vi "Wave Array Record LV2.vi"(2 "吸声测试结果IN":T1, 3 "W / R":enum16{"Write", "Read"}(ring)) -> (0 "吸声测试结果Out":T1)   [LabVIEW 2018]
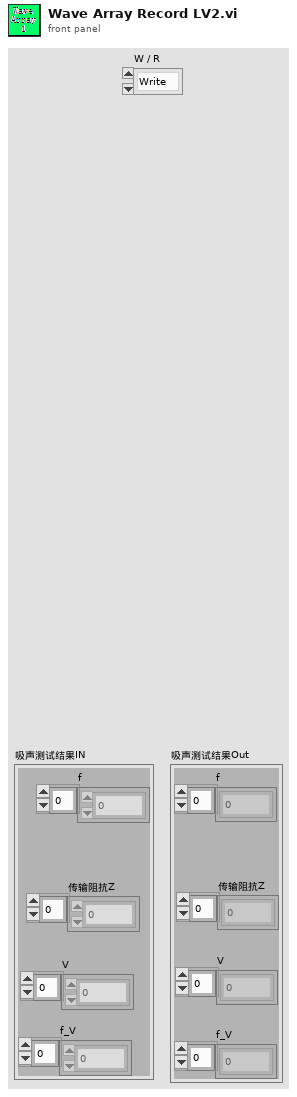
[diagram p1: front panel]
types:
  T1 = cluster{"f":dbl[], "传输阻抗Z":cdb[], "V":cdb[], "f_V":dbl[]}
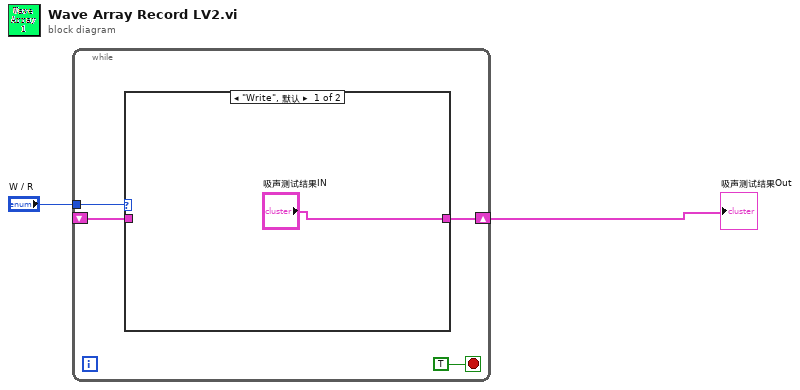
[diagram p0: block diagram]
diagram:
  n1 = while {
    tunnel: "W / R" -> [w5]
    shift-right: [w4] -> w1
    shift-left: _ -> [w3]
    stop <- TRUE stop-if-true
    n2 = case shown="\"Write\", 默认" w5 {
      tunnel: ["吸声测试结果IN" w8] -> w4
      tunnel: w3 -> [_ w8]
      frame "Write", Default {
      }
      frame "Read" {
      }
    }
  }
  "吸声测试结果Out" <- w1
